vi "TSCAN SetMapping.vi"(0 "路径输入":path, 7 "Tsapp_set_mapping_verbose_Type":T1={"AAppChannelType"=0, "AAppChannel"=0, "AHardwareType"=3, "AHardwareSubType"=3, "HardwareIndex"=0, "AHardwareChannel"=0, "AEnableMapping"=1, "ABaudrateKbps"=500.0, "AListenOnly"=0, "Int120Ohm"=1} {"Int120Ohm" items=["Disable", "Enable"]; "AListenOnly" items=["Normal", "ListenOnly"]; "ABaudrateKbps" format="%#_g  k"; "AEnableMapping" items=["Disable", "Enable"]; "AAppChannelType" items=["APP_CAN", "APP_LIN"]; "AHardwareChannel" items=["CHN1", "CHN2", "CHN3", "CHN4", "CHN5", "CHN6", "CHN7", "CHN8", "CHN9", "CHN10", "CHN11", "CHN12", "CHN13", "CHN14", "CHN15", "CHN16", "CHN17", "CHN18", "CHN19", "CHN20", "CHN21", "CHN22", "CHN23", "CHN24", "CHN25", "CHN26", "CHN27", "CHN28", "CHN29", "CHN30", "CHN31", "CHN32"]; "AAppChannel" items=["CHN1", "CHN2", "CHN3", "CHN4", "CHN5", "CHN6", "CHN7", "CHN8", "CHN9", "CHN10", "CHN11", "CHN12", "CHN13", "CHN14", "CHN15", "CHN16", "CHN17", "CHN18", "CHN19", "CHN20", "CHN21", "CHN22", "CHN23", "CHN24", "CHN25", "CHN26", "CHN27", "CHN28", "CHN29", "CHN30", "CHN31", "CHN32"]; "AHardwareType" items=["BUS_UNKNOWN_TYPE", "TS_TCP_DEVICE", "XL_USB_DEVICE", "TS_USB_DEVICE", "PEAK_USB_DEVICE", "KVASER_USB_DEVICE", "ZLG_USB_DEVICE", "ICS_USB_DEVICE", "TS_TC1005_DEVICE"]; "AHardwareSubType" items=["TS_UNKNOWN_DEVICE", "TSCAN_PRO", "TSCAN_Litel", "TC1001", "TL1001", "TC1011", "TSInterface", "TC1002", "TC1014"]}, 11 "错误输入（无错误）":errorcluster) -> (4 "路径输出":path, 15 "错误输出":errorcluster)   [LabVIEW 2013]
panel:
  in  "CANCount":i32(ring)=1 items=["1通道"=1, "2通道"=2, "3通道"=3, "4通道"=4, "5通道"=5]
  out "Set_Baudrated_Successfully":bool
  out "Mapping_Successfully":bool
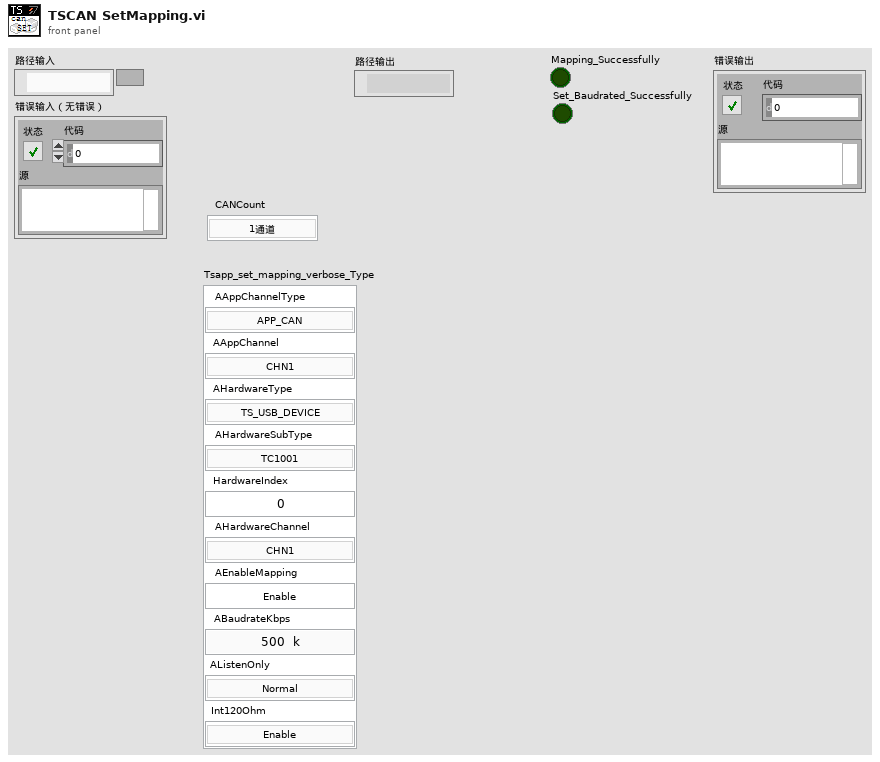
[diagram p1: front panel]
types:
  T1 = cluster{"AAppChannelType":i32, "AAppChannel":i32, "AHardwareType":i32, "AHardwareSubType":i32, "HardwareIndex":i32, "AHardwareChannel":i32, "AEnableMapping":u32, "ABaudrateKbps":sgl, "AListenOnly":u32, "Int120Ohm":u32}
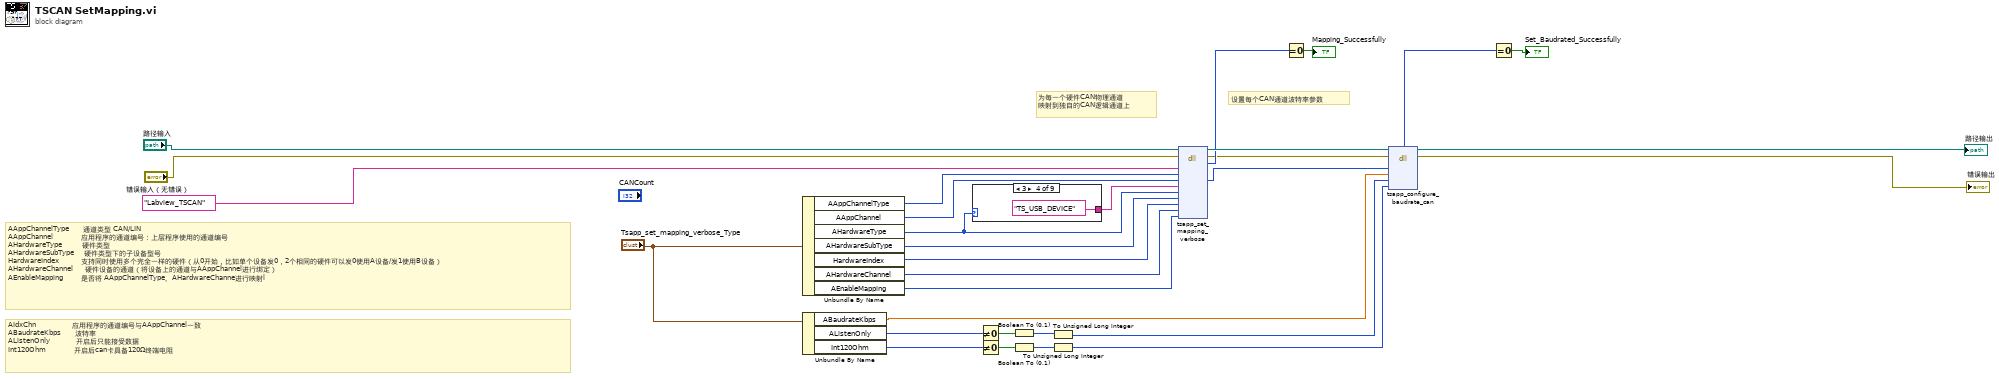
[diagram p0: block diagram]
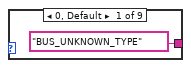
[diagram p2: hidden frame]
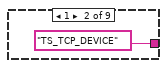
[diagram p3: hidden frame]
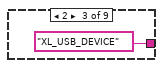
[diagram p4: hidden frame]
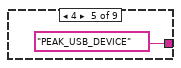
[diagram p5: hidden frame]
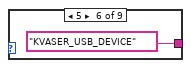
[diagram p6: hidden frame]
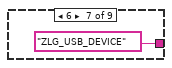
[diagram p7: hidden frame]
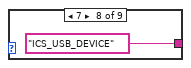
[diagram p8: hidden frame]
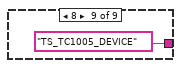
[diagram p9: hidden frame]
diagram:
  # "设置每个CAN通道波特率参数"
  # "为每一个硬件CAN物理通道\n映射到独自的CAN逻辑通道上"
  # "AIdxChn                  应用程序的通道编号与AAppChannel一致\nABaudrateKbps       波特率\nAListenOnly             开启后只能接受数据\nInt120Ohm              开启后can卡具备120Ω终端电阻"
  # "AAppChannelType       通道类型 CAN/LIN\nAAppChannel              应用程序的通道编号：上层程序使用的通道编号\nAHardwareType          硬件类型\nAHardwareSubType     硬件类型下的子设备型号\nHardwareIndex           支持同时使用多个完全一样的硬件（从0开始，比如单个设备发0，2个相同的硬件可以发0使用A设备/发1使用B设备）\nAHardwareChannel      硬件设备的通道（将设备上的通道与AAppChannel进行绑定）\nAEnableMapping         是否将 AAppChannelType、AHardwareChanne进行映射l"
  n1 = Unbundle By Name("Tsapp_set_mapping_verbose_Type") -> ("AAppChannelType"=w13:i32, "AAppChannel"=w12:i32, "AHardwareType"=w11:i32, "AHardwareSubType"=w10:i32, "HardwareIndex"=w9:i32, "AHardwareChannel"=w8:i32, "AEnableMapping"=w7:u32)
  n2 = Unbundle By Name("Tsapp_set_mapping_verbose_Type") -> ("ABaudrateKbps"=w6:sgl, "AListenOnly"=w5:u32, "Int120Ohm"=w4:u32)
  n3 = case shown="3" w11 {
    tunnel: ["BUS_UNKNOWN_TYPE" ("AHardwareName") "TS_TCP_DEVICE" ("AHardwareName") "XL_USB_DEVICE" ("AHardwareName") "TS_USB_DEVICE" ("AHardwareName") "PEAK_USB_DEVICE" ("AHardwareName") "KVASER_USB_DEVICE" ("AHardwareName") "ZLG_USB_DEVICE" ("AHardwareName") "ICS_USB_DEVICE" ("AHardwareName") "TS_TC1005_DEVICE" ("AHardwareName")] -> w24
    frame 0, Default {
    }
    frame 1 {
    }
    frame 2 {
    }
    frame 3 {
    }
    frame 4 {
    }
    frame 5 {
    }
    frame 6 {
    }
    frame 7 {
    }
    frame 8 {
    }
  }
  n4 = Not Equal To 0?(x=w5) -> (x != 0?=w23:bool)
  n5 = Not Equal To 0?(x=w4) -> (x != 0?=w22:bool)
  n6 = Boolean To (0,1)(Boolean=w23) -> (0, 1=w17:i16)
  n7 = Boolean To (0,1)(Boolean=w22) -> (0, 1=w16:i16)
  n8 = To Unsigned Long Integer(number=w17) -> (unsigned 32bit integer=w14:u32)
  n9 = To Unsigned Long Integer(number=w16) -> (unsigned 32bit integer=w15:u32)
  n10 = dll-call lib="PTH1Habs CUsers\nAdministratorDesktopTS_Can通讯PathTSMaster.dll" fn="tsapp_set_mapping_verbose"(path in="路径输入", error in="错误输入（无错误）", "FAPppName"="Labview_TSCAN" ("AppName"), "AChnType"=w13, "FAppChannelIndex"=w12, "AHWDeviceName"=w24, "AHWDeviceType"=w11, "AHWDeviceSubType"=w10, "AldHW"=w9, "AldHWChn"=w8, "FMappingDisabled"=w7) -> (path out=w25:path, error out=w19:errorcluster, "tsapp_set_mapping_verbose"=w20:i32, "FAppChannelIndex"=w18:i32)  [unwired: 9 in]
  n11 = Equal To 0?(x=w20) -> (x = 0?=→"Mapping_Successfully":bool)
  n12 = dll-call lib="PTH1Habs CUsers\nAdministratorDesktopTS_Can通讯PathTSMaster.dll" fn="tsapp_configure_baudrate_can"(path in=w25, error in=w19, "ALdxChn"=w18, "ABaudrateKbps"=w6, "AlistenOnly"=w14, "AlnstallTermResistor120Ohm"=w15) -> (path out=→"路径输出":path, error out=→"错误输出":errorcluster, "tsapp_configure_baudrate_can"=w29:i32)  [unwired: 5 in]
  n13 = Equal To 0?(x=w29) -> (x = 0?=→"Set_Baudrated_Successfully":bool)
